vi "CompareVersions.vi"(8 "error in (no error)":errorcluster) -> (0 "error out":errorcluster, 2 "FileVersion":string, 3 "Web File Version":string)   [LabVIEW 2013, in "main.lvlib"]
uses:
  main.lvlib
  <vilib>/httpClient/LabVIEWHTTPClient.lvlib
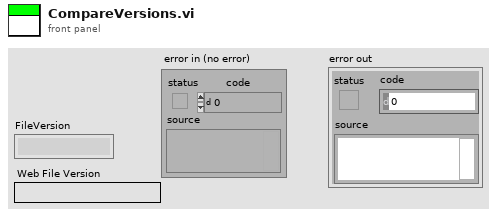
[diagram p1: front panel]
types:
  T1 = typedef "LabVIEWHTTPClient.lvlib/ClientHandle.ctl" = refnum<k1>
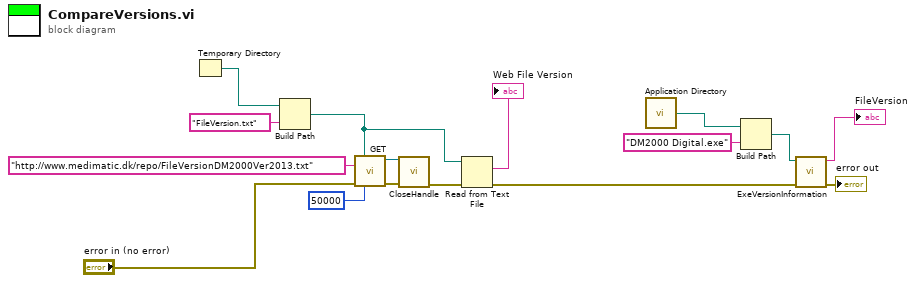
[diagram p0: block diagram]
diagram:
  n1 = Temporary Directory() -> (w4:path)
  n2 = Build Path(base path=w4, name or relative path="FileVersion.txt") -> (appended path=w3:path)
  n3 = call <vilib>:"GET.vi"("output file"=w3, "url"="http://www.medimatic.dk/repo/FileVersionDM2000Ver2013.txt", "error in (no error)"="error in (no error)", "timeout (10000)"=50000) -> ("client handle out"=w8:T1, "error out"=w7:errorcluster)  [unwired: 8 in, 2 out]
  n4 = call <vilib>:"CloseHandle.vi"("client handle"=w8, "error in (no error)"=w7) -> ("error out"=w5:errorcluster)  [unwired: 13 in]
  n5 = Read from Text File(file (use dialog)=w3, error in=w5) -> (text=→"Web File Version":string, error out=w12:errorcluster)  [unwired: 2 in, 2 out]
  n6 = call <vilib>:"Application Directory.vi"() -> ("Application Directory"=w15:path)
  n7 = Build Path(base path=w15, name or relative path="DM2000 Digital.exe") -> (appended path=w13:path)
  n8 = call "ExeVersionInformation.vi"("error in (no error)"=w12, "path"=w13) -> ("error out"=→"error out":errorcluster, "FileVersion"=→"FileVersion":string)  [unwired: 8 in]
